vi "Calculate Per-Site Trim ROUT.vi"(0 "Per Site ROUT In":u8[](array[numeric]) format="%08b", 5 "Per-Site Cur Sensitivity(dBV)":dbl[](array[numeric]), 7 "Target Sensitivity(dBV)":dbl, 9 "Trim Method":T1, 11 "error in (no error)":errorcluster) -> (4 "Per Site ROUT Out":u8[](array[numeric]) format="%08b", 6 "Per-Site Sensitivity Post Trim estimate (dBV)":dbl[](array[numeric]), 15 "error out":errorcluster)   [LabVIEW 2020]
uses:
  Trim Method Enum.ctl
  bf466052-ea92-4a45-82bc-ac32980f6788.vi
  c19c1bd3-1f45-4ff3-88d9-50e99dbf744e.vi
  327cd94f-b653-424f-8c8e-98dce99e9d80.vi
  7bf12a61-7b83-403b-af7f-35e46ed71a3d.vi
  8fd79813-1e20-4522-8fb0-3fc4d3ca482c.vi
  a4955629-fc07-47e2-9e63-39cb8948916b.vi
  e6f8d5c4-e4ba-483e-b8ab-181baf4eb14a.vi
  1c37a866-eb25-4279-bf54-2b2d87927dad.vi
  41b9e9b2-5d2f-4353-a293-58e30c274a90.vi
  Gain Lookup Table.vi
  <vilib>/gmath/interp.llb/Interpolate 1D.vi
  Vbias Gain Lookup Table.vi
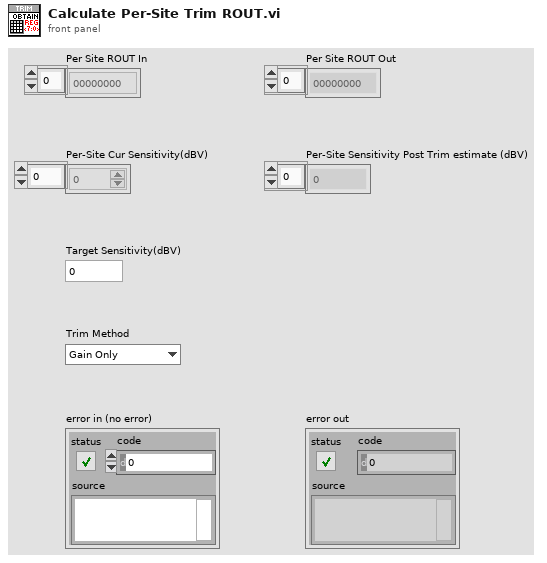
[diagram p1: front panel]
types:
  T1 = typedef "Trim Method Enum.ctl" = enum16{"Gain Only", "Gain then Vbias", "Gain Vbias Combo"}
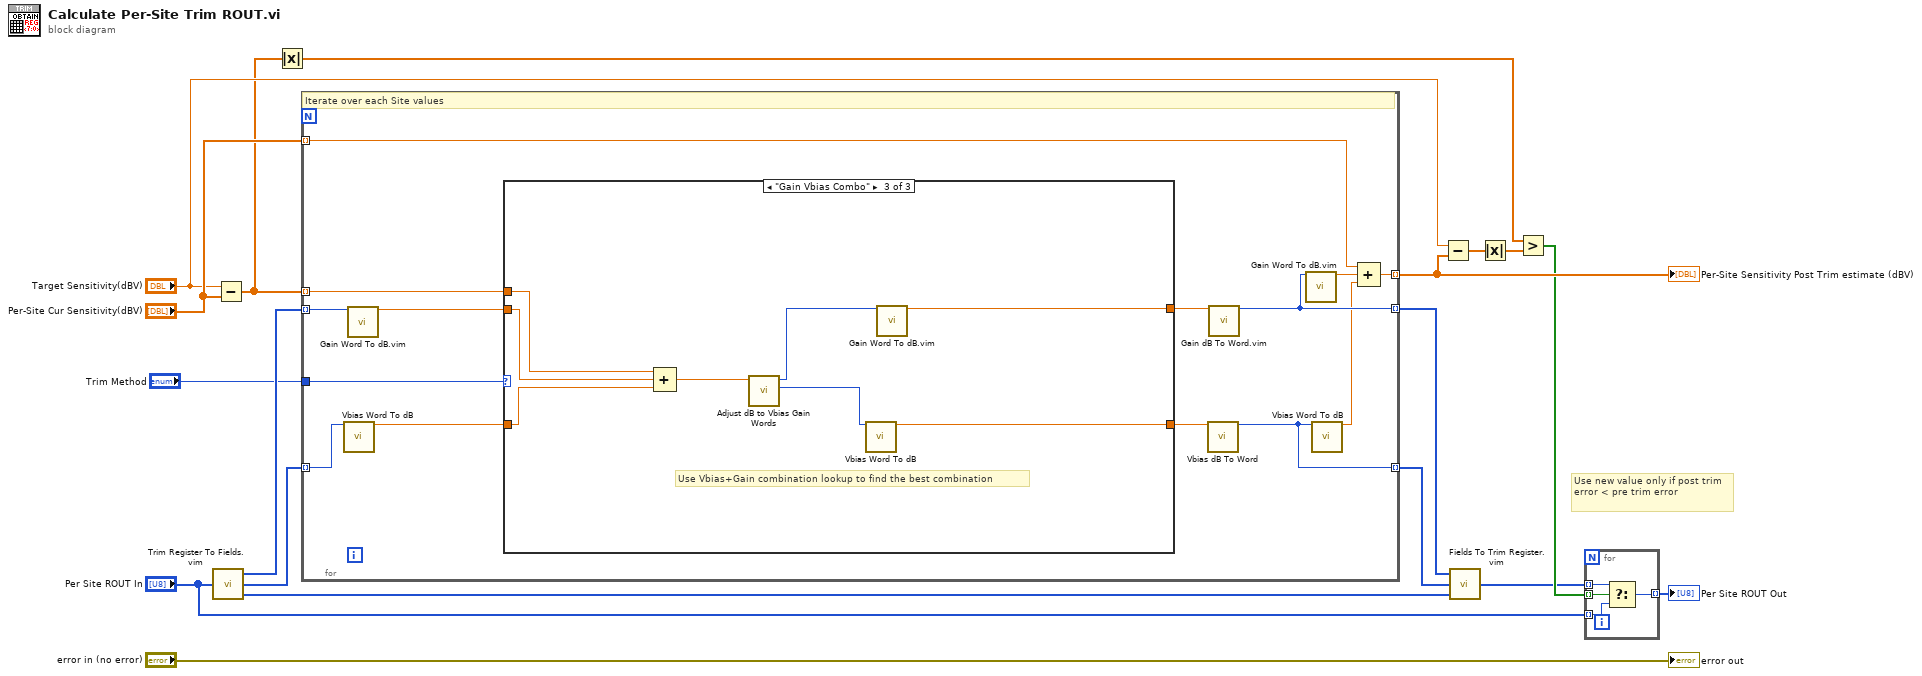
[diagram p0: block diagram]
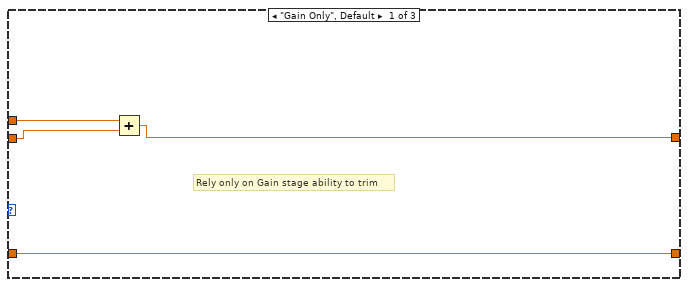
[diagram p2: hidden frame]
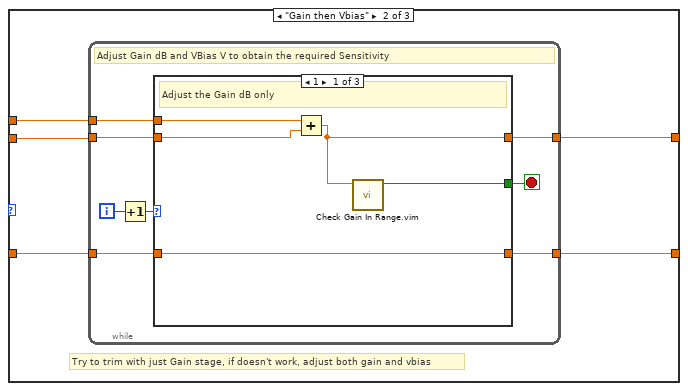
[diagram p3: hidden frame]
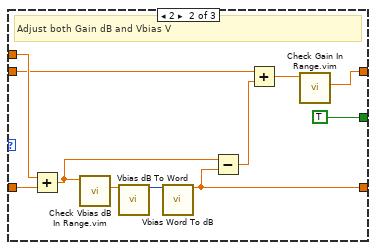
[diagram p4: hidden frame]
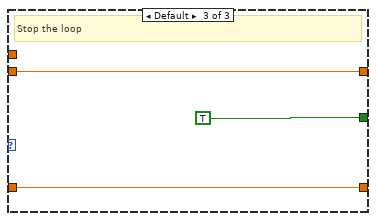
[diagram p5: hidden frame]
diagram:
  # "Use new value only if post trim error < pre trim error"
  n1 = call "Trim Register To Fields.vim"("ROUT"="Per Site ROUT In") -> ("Mode"=w15:u8[], "Vbias"=w16:u8[], "Gain"=w18:u8[])  [unwired: 2 in]
  n2 = Subtract(x="Target Sensitivity(dBV)", y="Per-Site Cur Sensitivity(dBV)") -> (x-y=w8:dbl[])
  n3 = Absolute Value(x=w8) -> (abs(x)=w6:dbl[])
  n4 = for {
    tunnel: w18 -> [w32] mode=indexing
    tunnel: w16 -> [w30] mode=indexing
    tunnel: w8 -> [w31] mode=indexing
    tunnel: [w28] -> w14 mode=indexing
    tunnel: [w29] -> w13 mode=indexing
    tunnel: "Per-Site Cur Sensitivity(dBV)" -> [w25] mode=indexing
    tunnel: [w24] -> w11 mode=indexing
    tunnel: "Trim Method" -> [w19]
    # "Iterate over each Site values"
    n5 = call "Vbias Word To dB.vi"("Vbias Word"=w30) -> ("dB"=w21:dbl)  [unwired: 14 in]
    n6 = call "Gain Word To dB.vim"("Gain Word"=w32) -> ("Gain dB"=w23:dbl)  [unwired: 14 in]
    n7 = case shown="\"Gain Vbias Combo\"" w19 {
      tunnel: w31 -> [w36 w41 w76]
      tunnel: w23 -> [w35 w40 w75]
      tunnel: [w34 w39 w69] -> w22
      tunnel: w21 -> [w33 w38 w74]
      tunnel: [w33 w37 w70] -> w20
      frame "Gain Only", Default {
        # "Rely only on Gain stage ability to trim"
        n8 = Add(x=w36, y=w35) -> (x+y=w34:dbl)
      }
      frame "Gain then Vbias" {
        # "Try to trim with just Gain stage, if doesn't work, adjust both gain and vbias"
        n9 = while {
          tunnel: w41 -> [w48]
          tunnel: w40 -> [w49]
          tunnel: [w47] -> w39
          tunnel: w38 -> [w43]
          tunnel: [w42] -> w37
          i -> [w46]
          stop <- w44 stop-if-true
          # "Adjust Gain dB and VBias V to obtain the required Sensitivity"
          n10 = Increment(x=w46) -> (x+1=w45:i32)
          n11 = case shown="1" w45 {
            tunnel: w49 -> [w54 w62 w67]
            tunnel: w48 -> [w53 w65 _]
            tunnel: [w52 w61 w67] -> w47
            tunnel: [w51 TRUE ("In Range?") TRUE] -> w44
            tunnel: w43 -> [w50 w58 w66]
            tunnel: [w50 w55 w66] -> w42
            frame 1 {
              # "Adjust the Gain dB only"
              n12 = Add(x=w53, y=w54) -> (x+y=w52:dbl)
              n13 = call "Check Gain In Range.vim"("Gain dB"=w52) -> ("In Range?"=w51:bool)  [unwired: 9 in, 1 out]
            }
            frame 2 {
              # "Adjust both Gain dB and Vbias V"
              n14 = Add(x=w65, y=w58) -> (x+y=w63:dbl)
              n15 = call "Check Vbias dB In Range.vim"("Vbias dB"=w63) -> ("Coerced Vbias dB"=w56:dbl)  [unwired: 9 in, 1 out]
              n16 = call "Vbias dB To Word.vi"("dB"=w56) -> ("Vbias Word"=w57:u8)  [unwired: 14 in]
              n17 = call "Vbias Word To dB.vi"("Vbias Word"=w57) -> ("dB"=w55:dbl)  [unwired: 14 in]
              n18 = Subtract(x=w63, y=w55) -> (x-y=w59:dbl)
              n19 = Add(x=w62, y=w59) -> (x+y=w64:dbl)
              n20 = call "Check Gain In Range.vim"("Gain dB"=w64) -> ("coerced Gain dB"=w61:dbl)  [unwired: 9 in, 1 out]
            }
            frame Default {
              # "Stop the loop"
            }
          }
        }
      }
      frame "Gain Vbias Combo" {
        # "Use Vbias+Gain combination lookup to find the best combination"
        n21 = Compound Arithmetic op=ADD(w76, w75, w74) -> (w73:dbl)
        n22 = call "Adjust dB to Vbias Gain Words.vi"("Adjust dB"=w73) -> ("Vbias Word"=w71:u8, "Gain Word"=w72:u8)  [unwired: 9 in]
        n23 = call "Vbias Word To dB.vi"("Vbias Word"=w71) -> ("dB"=w70:dbl)  [unwired: 14 in]
        n24 = call "Gain Word To dB.vim"("Gain Word"=w72) -> ("Gain dB"=w69:dbl)  [unwired: 14 in]
      }
    }
    n25 = call "Vbias dB To Word.vi"("dB"=w20) -> ("Vbias Word"=w28:u8)  [unwired: 14 in]
    n26 = call "Gain dB To Word.vim"("Gain dB"=w22) -> ("Gain Word"=w29:u8)  [unwired: 14 in]
    n27 = call "Gain Word To dB.vim"("Gain Word"=w29) -> ("Gain dB"=w27:dbl)  [unwired: 14 in]
    n28 = call "Vbias Word To dB.vi"("Vbias Word"=w28) -> ("dB"=w26:dbl)  [unwired: 14 in]
    n29 = Compound Arithmetic op=ADD(w25, w27, w26) -> (w24:dbl)
  }
  "Per-Site Sensitivity Post Trim estimate (dBV)" <- w11
  n30 = Subtract(x="Target Sensitivity(dBV)", y=w11) -> (x-y=w9:dbl[])
  n31 = call "Fields To Trim Register.vim"("Mode"=w15, "Vbias"=w14, "Gain"=w13) -> ("ROUT"=w4:u8[])  [unwired: 2 in]
  n32 = Absolute Value(x=w9) -> (abs(x)=w7:dbl[])
  n33 = Greater?(x=w6, y=w7) -> (0:w5:bool[])
  n34 = for {
    tunnel: w5 -> [w80] mode=indexing
    tunnel: w4 -> [w79] mode=indexing
    tunnel: "Per Site ROUT In" -> [w78] mode=indexing
    tunnel: [w77] -> w2 mode=indexing
    n35 = Select(t=w79, s=w80, f=w78) -> (s? t:f=w77:u8)
  }
  "Per Site ROUT Out" <- w2
  "error out" <- "error in (no error)"
